vi "Helper.vi"(1 "tsRef":refnum<vi>, 2 "op":T2(ring)=enum."deploy", 3 "instVIref":T1) -> (0 "status":u64)   [LabVIEW 2020, in "NI_TargetHelper.lvlib"]
uses:
  <vilib>/TargetSupport/NI_TargetHelper/NI_TargetHelper.lvlib
  <vilib>/TargetSupport/NI_TargetHelper/Instance VIref.ctl
  <vilib>/TargetSupport/NI_TargetHelper/Base Target/Base Target.lvclass
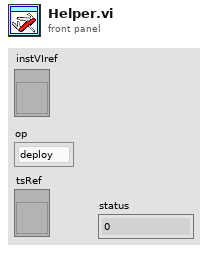
[diagram p1: front panel]
types:
  T1 = typedef "NI_TargetHelper.lvlib/Instance VIref.ctl" = refnum<vi>
  T2 = enum16{"status", "update", "compile", "deploy", "run", "stop", "init"}
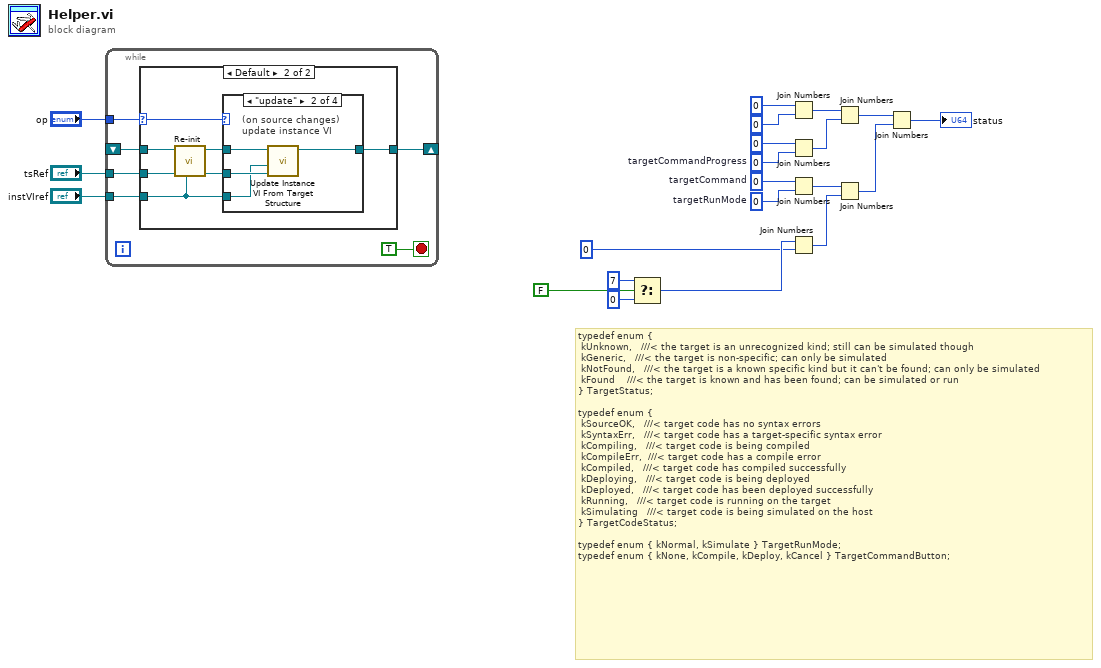
[diagram p0: block diagram]
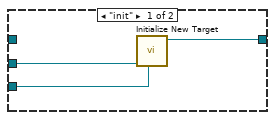
[diagram p2: hidden frame]
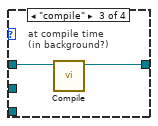
[diagram p4: hidden frame]
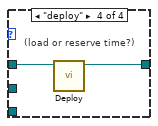
[diagram p5: hidden frame]
diagram:
  w12 = u8 0  # targetCommandProgress
  w19 = u8 0  # targetCommand
  w18 = u8 0  # targetRunMode
  # "typedef enum {\n\tkUnknown,\t\t\t///< the target is an unrecognized kind; still can be simulated though\n\tkGeneric,\t\t\t///< the target is non-specific; can only be simulated\n\tkNotFound,\t\t\t///< the target is a known specific kind but it can't be found; can only be simulated\n\tkFound\t\t\t\t///< the target is known and has been found; can be simulated or run\n} TargetStatus;\n\ntypedef enum {\n\tkSourceOK,\t\t\t///< target code has no syntax errors\n\tkSyntaxErr,\t\t\t///< target code has a target-specific syntax error\n\tkCompiling,\t\t\t///< target code is being compiled\n\tkCompileErr,\t\t///< target code has a compile error\n\tkCompiled,\t\t\t///< target code has compiled successfully\n\tkDeploying,\t\t\t///< target code is being deployed\n\tkDeployed,\t\t\t///< target code has been deployed successfully\n\tkRunning,\t\t\t///< target code is running on the target\n\tkSimulating\t\t\t///< target code is being simulated on the host\n} TargetCodeStatus;\n\ntypedef enum { kNormal, kSimulate } TargetRunMode;\ntypedef enum { kNone, kCompile, kDeploy, kCancel } TargetCommandButton;"
  n1 = while {
    tunnel: "op" -> [w27]
    tunnel: "instVIref" -> [w26]
    tunnel: "tsRef" -> [w25]
    shift-right: [w23] -> _
    shift-left: _ -> [w22]
    stop <- TRUE stop-if-true
    n2 = case shown="Default" w27 {
      selector: w27 -> [_ w37]
      tunnel: w26 -> [w30 w33]
      tunnel: w25 -> [w29 w32]
      tunnel: [w28 w36] -> w23
      tunnel: w22 -> [_ w35]
      frame "init" {
        n3 = call <vilib>:"Initialize New Target.vi"("instVIref"=w30, "tsRef"=w29) -> ("target out"=w28:refnum<class "Base Target.lvclass">)  [unwired: 9 in]
      }
      frame Default {
        n4 = call-dynamic "Re-init.vi"("instVIref"=w33, "tsRef"=w32, "target in"=w35) -> ("tsRef out"=w31:refnum<vi>, "target out"=w34:refnum<class "Base Target.lvclass">)  [unwired: 7 in]
        n5 = case shown="\"update\"" w37 {
          tunnel: w33 -> [_ w39 _ _]
          tunnel: w31 -> [_ w42 _ _]
          tunnel: [w38 w41 w43 w45] -> w36
          tunnel: w34 -> [w38 w40 w44 w46]
          frame Default {
          }
          frame "update" {
            # "(on source changes)\nupdate instance VI"
            n6 = call <vilib>:"Update Instance VI From Target Structure.vi"("tsRef"=w42, "instVIref"=w39, "target in"=w40) -> ("target out"=w41:refnum<class "Base Target.lvclass">)  [unwired: 8 in]
          }
          frame "compile" {
            # "at compile time\n(in background?)"
            n7 = call-dynamic "Compile.vi"("target in"=w44) -> ("target out"=w43:refnum<class "Base Target.lvclass">)  [unwired: 10 in]
          }
          frame "deploy" {
            # "(load or reserve time?)"
            n8 = call-dynamic "Deploy.vi"("target in"=w46) -> ("target out"=w45:refnum<class "Base Target.lvclass">)  [unwired: 10 in]
          }
        }
      }
    }
  }
  n9 = Select(t=u8 7, s=FALSE, f=u8 0) -> (s? t:f=w3:u8)
  n10 = Join Numbers(hi=u8 0, lo=u8 0) -> ((hi.lo)=w14:u16)
  n11 = Join Numbers(hi=u8 0, lo=w12) -> ((hi.lo)=w13:u16)
  n12 = Join Numbers(hi=w19, lo=w18) -> ((hi.lo)=w16:u16)
  n13 = Join Numbers(hi=w3, lo=u8 0) -> ((hi.lo)=w17:u16)
  n14 = Join Numbers(hi=w14, lo=w13) -> ((hi.lo)=w8:u32)
  n15 = Join Numbers(hi=w16, lo=w17) -> ((hi.lo)=w15:u32)
  n16 = Join Numbers(hi=w8, lo=w15) -> ((hi.lo)=→"status":u64)
